vi "get default name.vi"(8 "error in":errorcluster, 11 "PLTarget cRIO in":refnum<class "PLTarget cRIO.lvclass">) -> (0 "error out":errorcluster, 2 "default name":string, 3 "PLTarget cRIO out":refnum<class "PLTarget cRIO.lvclass">)   [LabVIEW 2013, in "PLTarget cRIO.lvclass"]
uses:
  PLTarget cRIO.lvclass
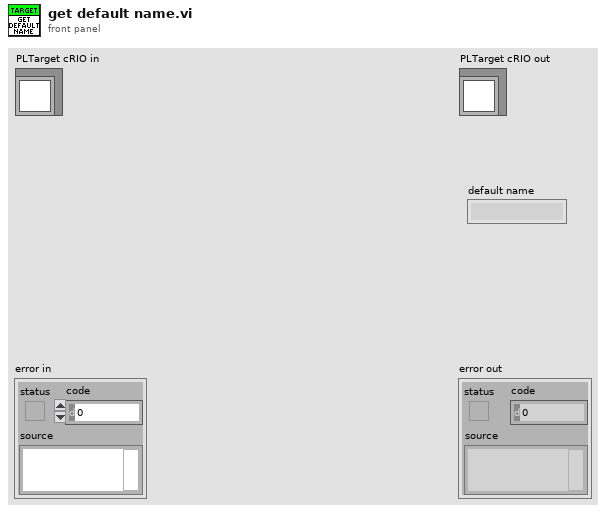
[diagram p1: front panel]
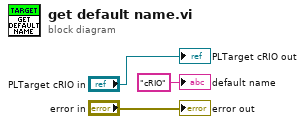
[diagram p0: block diagram]
diagram:
  "error out" <- "error in"
  "PLTarget cRIO out" <- "PLTarget cRIO in"
  "default name" <- "cRIO" ("default name")
